vi "StartTask.vi"(8 "error in (no error)":errorcluster, 11 "Task_Abstr in":refnum<class "Task_Abstr.lvclass">) -> (0 "error out":errorcluster, 3 "Task_Abstr out":refnum<class "Task_Abstr.lvclass">)   [LabVIEW 2025, in "Task_Abstr.lvlib" / "Task_Abstr.lvclass"]
uses:
  Task_Abstr.lvclass
  Task_Abstr.lvclass/Task_Abstr.ctl
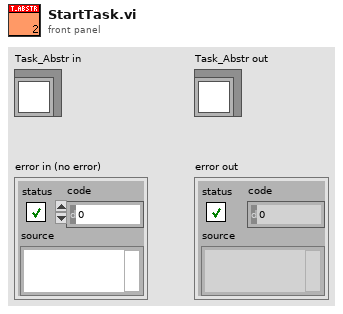
[diagram p1: front panel]
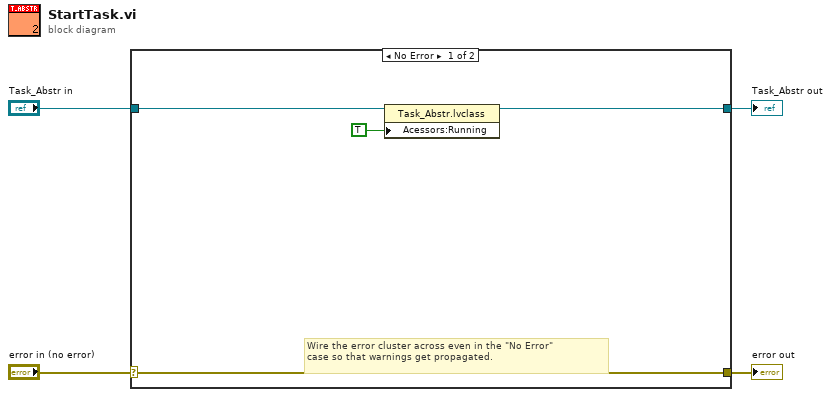
[diagram p0: block diagram]
diagram:
  n1 = case shown="No Error" "error in (no error)" {
    selector: "error in (no error)" -> [w8 w10]
    tunnel: [w8 w10] -> w3
    tunnel: [w5 w9] -> w1
    tunnel: "Task_Abstr in" -> [w6 w9]
    frame No Error {
      # "Wire the error cluster across even in the \"No Error\"\ncase so that warnings get propagated."
      n2 = property class="Task_Abstr.lvclass"(reference=w6, "Acessors:Running"=TRUE ("Running")) -> (reference out=w5:refnum<class "Task_Abstr.lvclass">)  [unwired: 1 in, 1 out]
    }
    frame Error {
    }
  }
  "error out" <- w3
  "Task_Abstr out" <- w1
